vi "Actor.vi"(9 "Actor Type":T1, 10 "Spawn":refnum<class "Spawn.lvclass">, 11 "Core Actor in":refnum<class "Core Actor.lvclass">) -> (0 "Error out":errorcluster, 3 "Core Actor out":refnum<class "Core Actor.lvclass">)   [LabVIEW 2025, in "jettl.lvlib" / "Actor.lvlib" / "Core Actor.lvclass"]
uses:
  Core Actor.lvclass
  Spawn/Spawn/Spawn.lvclass
  Core Actor.lvclass/Core Actor.ctl
  Actor Type.ctl
  Actor.lvlib
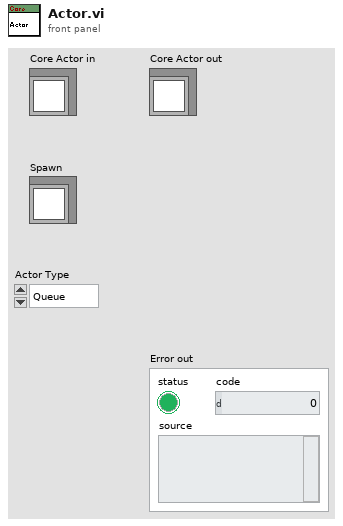
[diagram p1: front panel]
types:
  T1 = typedef "jettl.lvlib/Actor.lvlib/Actor Type.ctl" = enum16{"Queue", "Event", "Notifier"}
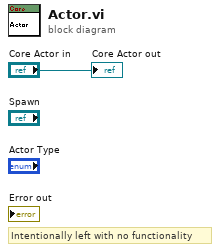
[diagram p0: block diagram]
diagram:
  # "Intentionally left with no functionality"
  "Core Actor out" <- "Core Actor in"
